vi "Master Control.vi"(11 "Enum":T1) -> ()   [LabVIEW 2014]
uses:
  SRE Enum.ctl
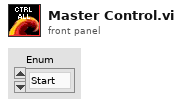
[diagram p1: front panel]
types:
  T1 = typedef "SRE Enum.ctl" = enum16{"Start", "Run", "End"}
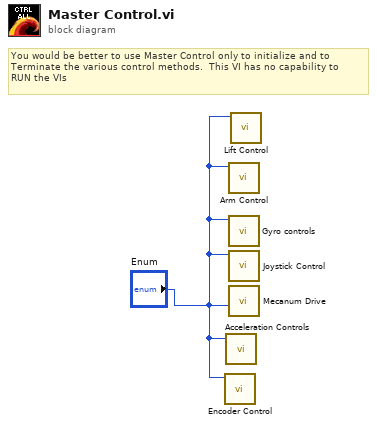
[diagram p0: block diagram]
diagram:
  # "You would be better to use Master Control only to initialize and to\nTerminate the various control methods.  This VI has no capability to\nRUN the VIs"
  n1 = call "Encoder Control.vi"("Enum"="Enum") -> ()  [unwired: 9 in, 2 out]
  n2 = call "Acceleration Controls.vi"("Enum"="Enum") -> ()  [unwired: 3 in, 1 out]
  n3 = call "Arm Control.vi"("Enum"="Enum") -> ()  [unwired: 10 in, 1 out]
  n4 = call "Gyro controls.vi"("Enum"="Enum") -> ()  [unwired: 10 in, 1 out]
  n5 = call "Joystick Control.vi"("Enum"="Enum") -> ()  [unwired: 9 in, 2 out]
  n6 = call "Mecanum Drive.vi"("Enum"="Enum") -> ()  [unwired: 11 in]
  n7 = call "Lift Control.vi"("Enum"="Enum") -> ()  [unwired: 10 in, 1 out]
